vi "viServerHostAccess_HostEntriesToHostNamesAndSymbols.vi"(0 "ACL in":refnum<k20>, 5 "principal array in":T1[](array[typedef]) {"principal"."ID"."b7" format="%02x"; "principal"."ID"."b6" format="%02x"; "principal"."ID"."b5" format="%02x"; "principal"."ID"."b4" format="%02x"; "principal"."ID"."b3" format="%02x"; "principal"."ID"."b2" format="%02x"; "principal"."ID"."b1" format="%02x"; "principal"."ID"."b0" format="%02x"; "principal"."ID"."b15" format="%02x"; "principal"."ID"."b14" format="%02x"; "principal"."ID"."b13" format="%02x"; "principal"."ID"."b12" format="%02x"; "principal"."ID"."b11" format="%02x"; "principal"."ID"."b10" format="%02x"; "principal"."ID"."b9" format="%02x"; "principal"."ID"."b8" format="%02x"; "domain"."ID"."b7" format="%02x"; "domain"."ID"."b6" format="%02x"; "domain"."ID"."b5" format="%02x"; "domain"."ID"."b4" format="%02x"; "domain"."ID"."b3" format="%02x"; "domain"."ID"."b2" format="%02x"; "domain"."ID"."b1" format="%02x"; "domain"."ID"."b0" format="%02x"; "domain"."ID"."b15" format="%02x"; "domain"."ID"."b14" format="%02x"; "domain"."ID"."b13" format="%02x"; "domain"."ID"."b12" format="%02x"; "domain"."ID"."b11" format="%02x"; "domain"."ID"."b10" format="%02x"; "domain"."ID"."b9" format="%02x"; "domain"."ID"."b8" format="%02x"}, 11 "error in (no error)":errorcluster) -> (4 "ACL out":refnum<k20>, 6 "principal array out":T1[](array[typedef]) {"principal"."ID"."b7" format="%02x"; "principal"."ID"."b6" format="%02x"; "principal"."ID"."b5" format="%02x"; "principal"."ID"."b4" format="%02x"; "principal"."ID"."b3" format="%02x"; "principal"."ID"."b2" format="%02x"; "principal"."ID"."b1" format="%02x"; "principal"."ID"."b0" format="%02x"; "principal"."ID"."b15" format="%02x"; "principal"."ID"."b14" format="%02x"; "principal"."ID"."b13" format="%02x"; "principal"."ID"."b12" format="%02x"; "principal"."ID"."b11" format="%02x"; "principal"."ID"."b10" format="%02x"; "principal"."ID"."b9" format="%02x"; "principal"."ID"."b8" format="%02x"; "domain"."ID"."b7" format="%02x"; "domain"."ID"."b6" format="%02x"; "domain"."ID"."b5" format="%02x"; "domain"."ID"."b4" format="%02x"; "domain"."ID"."b3" format="%02x"; "domain"."ID"."b2" format="%02x"; "domain"."ID"."b1" format="%02x"; "domain"."ID"."b0" format="%02x"; "domain"."ID"."b15" format="%02x"; "domain"."ID"."b14" format="%02x"; "domain"."ID"."b13" format="%02x"; "domain"."ID"."b12" format="%02x"; "domain"."ID"."b11" format="%02x"; "domain"."ID"."b10" format="%02x"; "domain"."ID"."b9" format="%02x"; "domain"."ID"."b8" format="%02x"}, 8 "Host names/addresses":string[](array[string]), 10 "Host access symbols":i32[](array[numeric]), 15 "error out":errorcluster)   [LabVIEW 2017]
uses:
  <vilib>/Platform/security/user/NI_Security Qualified Domain-Principal Pair.ctl
  <vilib>/Platform/security/user/NI_Security Domain.ctl
  <vilib>/Platform/security/user/NI_Security Identifier.ctl
  <vilib>/Platform/security/user/NI_Security Principal.ctl
  <vilib>/Platform/security/user/NI_Security PrincipalType.ctl
  <resource>/dialog/PreferencesDialog/PreferencePages/SharedPrefPage_SubVIs/ServerAccessGlyphSelector.ctl
  <vilib>/Platform/security/user/NI_Security AccessRights_CloseRef.vi
  <vilib>/Platform/security/user/NI_Security HostEntry_CloseRef.vi
  <resource>/objmgr/Security.rc
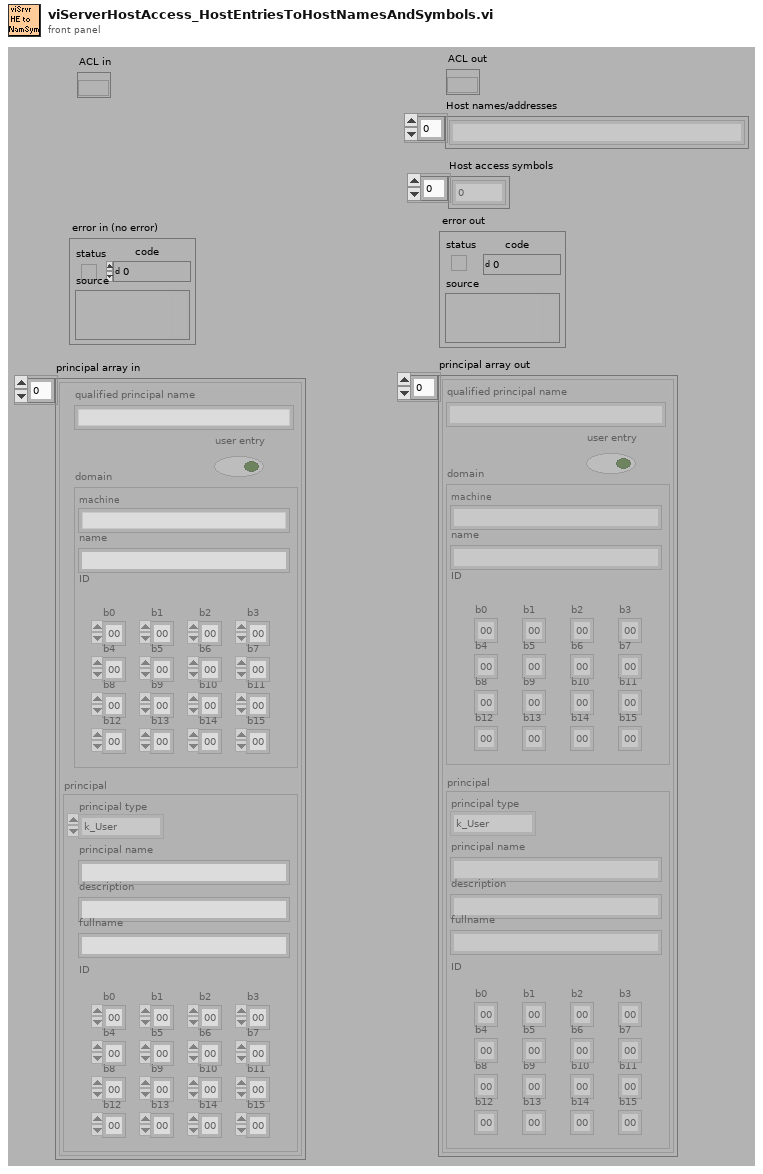
[diagram p1: front panel]
types:
  T1 = typedef "NI_Security Qualified Domain-Principal Pair.ctl" = cluster{"qualified principal name":string, "domain":T2, "principal":T4, "user entry":bool}
  T2 = typedef "NI_Security Domain.ctl" = cluster{"machine":string, "name":string, "ID":T3}
  T3 = typedef "NI_Security Identifier.ctl" = cluster{"b0":u8, "b1":u8, "b2":u8, "b3":u8, "b4":u8, "b5":u8, "b6":u8, "b7":u8, "b8":u8, "b9 ":u8, "b10":u8, "b11":u8, "b12":u8, "b13":u8, "b14":u8, "b15":u8}
  T4 = typedef "NI_Security Principal.ctl" = cluster{"principal type":T5, "principal name":string, "description":string, "fullname":string, "ID":T3}
  T5 = typedef "NI_Security PrincipalType.ctl" = enum16{"k_User", "k_Group"}
  T6 = typedef "ServerAccessGlyphSelector.ctl" = u16
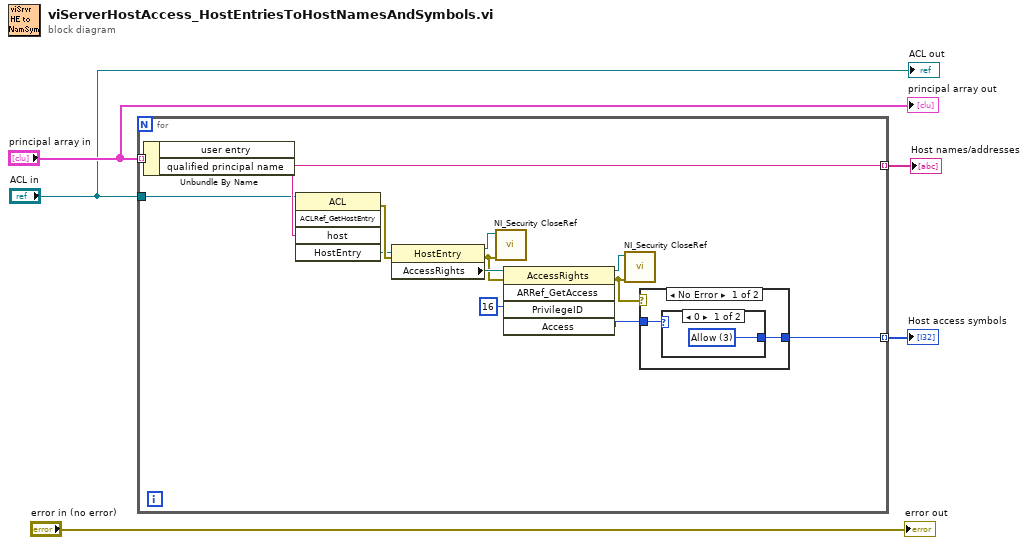
[diagram p0: block diagram]
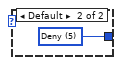
[diagram p2: hidden frame]
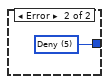
[diagram p3: hidden frame]
diagram:
  n1 = for {
    tunnel: "principal array in" -> [w18] mode=indexing
    tunnel: [w14] -> w3 mode=indexing
    tunnel: "ACL in" -> [w13]
    tunnel: [w6] -> w1 mode=indexing
    n2 = Unbundle By Name(w18) -> ("qualified principal name"=w14:string)  [unwired: 1 out]
    n3 = invoke class="ACL" method="ACLRef_GetHostEntry"(reference=w13, "host"=w14) -> (error out=w16:errorcluster, "HostEntry"=w15:refnum<k20>)  [unwired: 3 in, 3 out]
    n4 = property class="HostEntry"(reference=w15, error in=w16) -> (reference out=w17:refnum<k20>, error out=w7:errorcluster, "AccessRights"=w12:refnum<k20>)
    n5 = call-poly <vilib>:"NI_Security CloseRef.vi"("error in (no error)"=w7, "security refnum"=w17) -> ()  [unwired: 9 in, 1 out]
    n6 = invoke class="AccessRights" method="ARRef_GetAccess"(reference=w12, error in=w7, "PrivilegeID"=u32 16) -> (reference out=w10:refnum<k20>, error out=w9:errorcluster, "Access"=w8:u32)  [unwired: 2 in, 2 out]
    n7 = call-poly <vilib>:"NI_Security CloseRef.vi"("error in (no error)"=w9, "security refnum"=w10) -> ()  [unwired: 9 in, 1 out]
    n8 = case shown="No Error" w9 {
      tunnel: w8 -> [w20 _]
      tunnel: [w19 w23] -> w6
      frame No Error {
        n9 = case shown="0" w20 {
          tunnel: [w21 w22] -> w19
          frame 0 {
            w21 = T6 3 items=["None", "AllowAllow", "AllowAllowError", "Allow", "AllowError", "Deny", "DenyError"] ("Server Access Glyph Selector")
          }
          frame Default {
            w22 = T6 5 items=["None", "AllowAllow", "AllowAllowError", "Allow", "AllowError", "Deny", "DenyError"] ("Server Access Glyph Selector")
          }
        }
      }
      frame Error {
        w23 = T6 5 items=["None", "AllowAllow", "AllowAllowError", "Allow", "AllowError", "Deny", "DenyError"] ("Server Access Glyph Selector")
      }
    }
  }
  "Host names/addresses" <- w3
  "Host access symbols" <- w1
  "error out" <- "error in (no error)"
  "principal array out" <- "principal array in"
  "ACL out" <- "ACL in"
